vi "Servo Pulse Gen..vi"() -> ()   [LabVIEW 2015]
uses:
  Slide Servo.ctl
  Galobal variable_TI.vi
  Project Setup/Globle Variable/GR_Servo.vi
panel:
  in  "x":bool
  out "Enum":T1
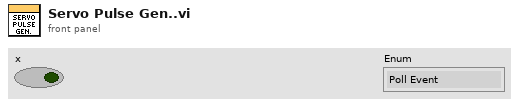
[diagram p1: front panel]
types:
  T1 = typedef "Slide Servo.ctl" = enum16{"Poll Event", "Servo CMD", "Slide Servo Home ", "Exit"}
  T2 = cluster{"Emergency_1":bool, "Reset_2":bool, "Air Pressure_4":bool, "Safety Sensor_5":bool, "Safety Sensor_6":bool, "Barcode Rev rs_24":bool, "Clamp fwd rs_21":bool, "Servo Fault":bool, "Home _3":bool}
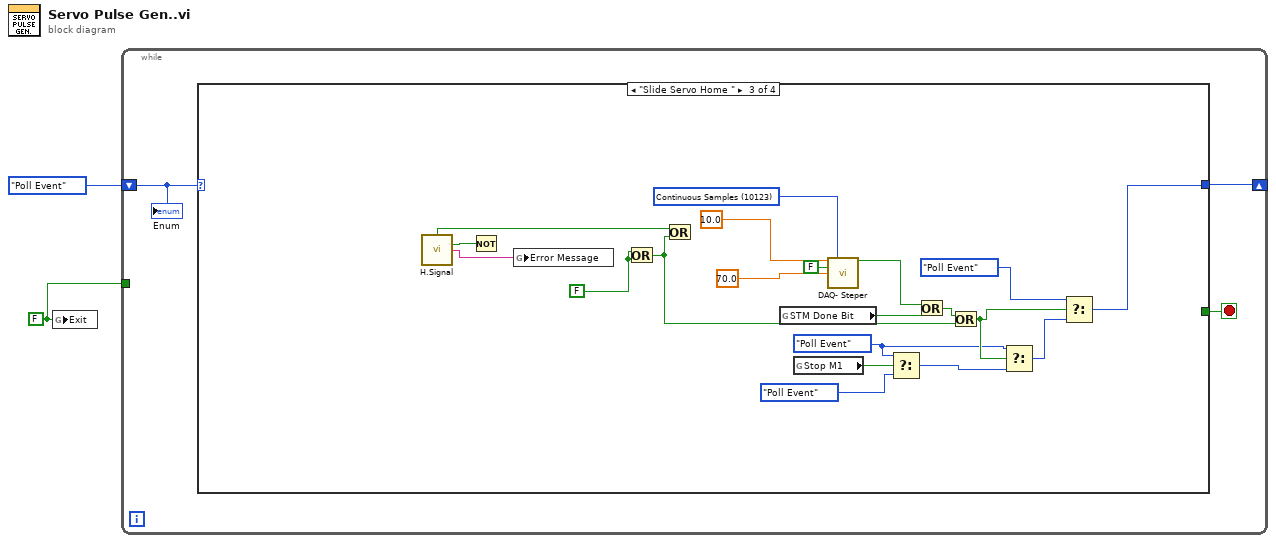
[diagram p0: block diagram]
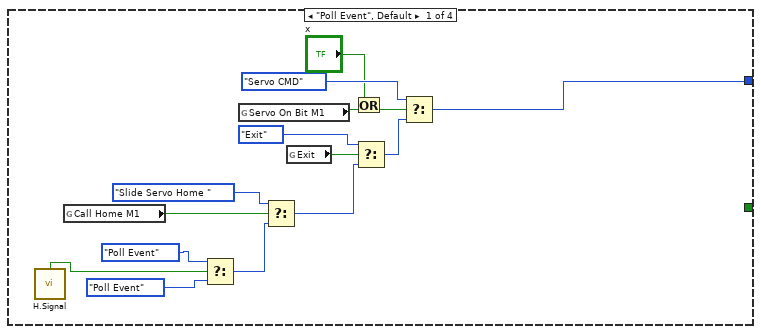
[diagram p2: hidden frame]
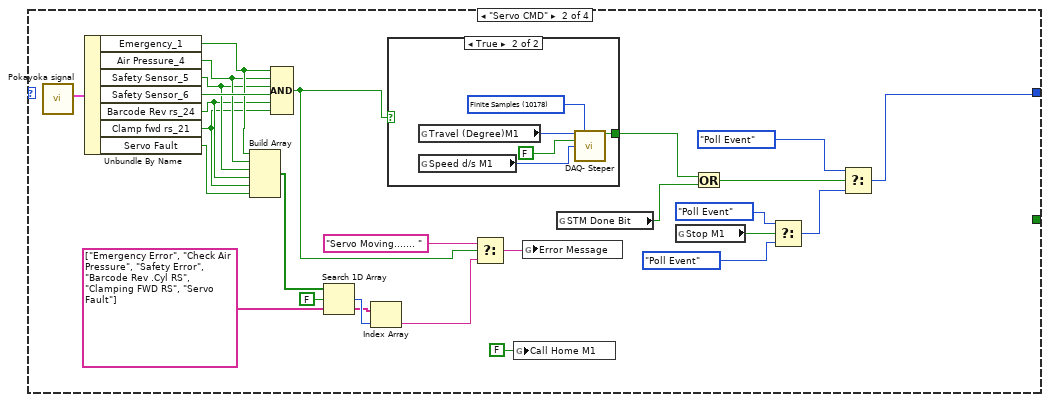
[diagram p3: hidden frame]
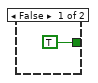
[diagram p4: hidden frame]
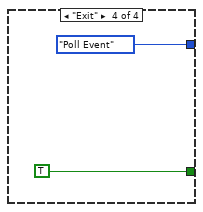
[diagram p5: hidden frame]
diagram:
  w1 = FALSE ("Exit")
  n1 = global write "Galobal variable_TI.vi" "Exit"(w1) -> ()
  n2 = while {
    shift-right: [w4] -> _
    shift-left: Slide_Servo."Poll Event" ("Enum") -> [w5]
    tunnel: w1 -> [_]
    stop <- w3 stop-if-true
    n3 = case shown="\"Slide Servo Home \"" w5 {
      tunnel: [w15 w42 w62 Slide_Servo."Poll Event" ("Enum")] -> w4
      tunnel: [_ _ _ TRUE] -> w3
      frame "Poll Event", Default {
        n4 = call "H.Signal.vi"() -> ("element"=w9:bool)  [unwired: 10 in, 5 out]
        n5 = global read "Galobal variable_TI.vi" "Call Home M1"() -> (w8:bool)
        n6 = Select(t=Slide_Servo."Poll Event" ("Enum"), s=w9, f=Slide_Servo."Poll Event" ("Enum")) -> (s? t:f=w11:T1)
        n7 = global read "GR_Servo.vi" "Servo On Bit M1"() -> (w18:bool)
        n8 = Select(t=Slide_Servo."Slide Servo Home " ("Enum"), s=w8, f=w11) -> (s? t:f=w13:T1)
        n9 = global read "Galobal variable_TI.vi" "Exit"() -> (w19:bool)
        n10 = Or(x="x", y=w18) -> (x .or. y?=w7:bool)
        n11 = Select(t=Slide_Servo."Exit" ("Enum"), s=w19, f=w13) -> (s? t:f=w20:T1)
        n12 = Select(t=Slide_Servo."Servo CMD" ("Enum"), s=w7, f=w20) -> (s? t:f=w15:T1)
      }
      frame "Servo CMD" {
        n13 = call "Pokayoka signal.vi"() -> ("output cluster"=w34:T2)  [unwired: 10 in, 1 out]
        n14 = Unbundle By Name(w34) -> ("Emergency_1"=w28:bool, "Air Pressure_4"=w27:bool, "Safety Sensor_5"=w26:bool, "Safety Sensor_6"=w33:bool, "Barcode Rev rs_24"=w25:bool, "Clamp fwd rs_21"=w24:bool, "Servo Fault"=w21:bool)
        n15 = Build Array(w28, w27, w26, w25, w24, w21) -> (w23:bool[])
        n16 = Compound Arithmetic op=AND(w28, w27, w26, w33, w25, w24) -> (w32:bool)
        n17 = Search 1D Array(1D array=w23, element=FALSE) -> (index of element=w31:i32)  [unwired: 1 in]
        n18 = Index Array(array=string[] ["Emergency Error", "Check Air Pressure", "Safety Error", "Barcode Rev .Cyl RS", "Clamping FWD RS", "Servo Fault"], index=w31) -> (element=w22:string)
        n19 = case shown="True" w32 {
          tunnel: [TRUE ("Task Done Bit") w50] -> w46
          frame False {
          }
          frame True {
            w48 = 10178 items=["Finite Samples"=10178, "Continuous Samples"=10123, "Hardware Timed Single Point"=12522] ("Mode")
            n20 = global read "GR_Servo.vi" "Travel (Degree)M1"() -> (w51:i32)
            n21 = global read "GR_Servo.vi" "Speed d/s M1"() -> (w52:i32)
            n22 = call "DAQ- Steper.vi"("Travel (Degree)"=w51, "Mode"=w48, "Home Condition"=FALSE, "Speed d/s"=w52) -> ("Task Done Bit"=w50:bool)  [unwired: 10 in, 1 out]
          }
        }
        n23 = Select(t="Servo Moving....... ", s=w32, f=w22) -> (s? t:f=w35:string)
        n24 = global write "Galobal variable_TI.vi" "Call Home M1"(FALSE ("Call Home M1")) -> ()
        n25 = global write "GR_Servo.vi" "Error Message"(w35) -> ()
        n26 = global read "Galobal variable_TI.vi" "STM Done Bit"() -> (w45:bool)
        n27 = global read "Galobal variable_TI.vi" "Stop M1"() -> (w41:bool)
        n28 = Or(x=w46, y=w45) -> (x .or. y?=w44:bool)
        n29 = Select(t=Slide_Servo."Poll Event" ("Enum"), s=w41, f=Slide_Servo."Poll Event" ("Enum")) -> (s? t:f=w38:T1)
        n30 = Select(t=Slide_Servo."Poll Event" ("Enum"), s=w44, f=w38) -> (s? t:f=w42:T1)
      }
      frame "Slide Servo Home " {
        w61 = 10123 items=["Finite Samples"=10178, "Continuous Samples"=10123, "Hardware Timed Single Point"=12522] ("Mode")
        w64 = Slide_Servo."Poll Event" ("Enum")
        w54 = FALSE ("y")
        n31 = call "H.Signal.vi"() -> ("element"=w55:bool, "HI Bit Auto"=w57:bool, "Error M Auto"=w58:string)  [unwired: 10 in, 3 out]
        n32 = Not(x=w57) -> ()  [unwired: 1 out]
        n33 = global write "GR_Servo.vi" "Error Message"(w58) -> ()
        n34 = Or(x=w54, y=w54) -> (x .or. y?=w56:bool)
        n35 = Or(x=w55, y=w56) -> ()  [unwired: 1 out]
        n36 = global read "Galobal variable_TI.vi" "STM Done Bit"() -> (w71:bool)
        n37 = global read "Galobal variable_TI.vi" "Stop M1"() -> (w68:bool)
        n38 = call "DAQ- Steper.vi"("Travel (Degree)"=10.0, "Mode"=w61, "Home Condition"=FALSE, "Speed d/s"=70.0) -> ("Task Done Bit"=w72:bool)  [unwired: 10 in, 1 out]
        n39 = Select(t=w64, s=w68, f=Slide_Servo."Poll Event" ("Enum")) -> (s? t:f=w65:T1)
        n40 = Or(x=w72, y=w71) -> (x .or. y?=w69:bool)
        n41 = Or(x=w69, y=w56) -> (x .or. y?=w66:bool)
        n42 = Select(t=w64, s=w66, f=w65) -> (s? t:f=w63:T1)
        n43 = Select(t=Slide_Servo."Poll Event" ("Enum"), s=w66, f=w63) -> (s? t:f=w62:T1)
      }
      frame "Exit" {
      }
    }
    "Enum" <- w5
  }
